vi "Coord window-Panel close handler.vi"   [LabVIEW 2017]
uses:
  Visualisation/Functional Imaging Viewer/SubVIs/Experiment header interface/Typedefs/Save-Load-Save as-Load last enum.ctl
  Globals/Coord window-Globals.vi
types:
  T1 = cluster{"Caption-Right button":string, "Caption-Left button":string, "Message to display":string, "Delay before close":u32, "Window Colour":u32, "Cancel button disabled?":enum8{"Enabled", "Disabled", "Disabled and Grayed Out"}}
  T2 = typedef "Coordinate list window refs.ctl" = cluster{"Window Name (i.e. Key)":string, "menu reference":refnum<k9>, "VI's reference":refnum<vi>, "Pane 1":refnum<vi>, "Pane 2":refnum<vi>, "Coord Listbox":refnum<vi>, "File name":refnum<vi>, "Picture Map":refnum<vi>, "Stage XYZ Position ind.":refnum<vi>}
  T3 = typedef "Save-Load-Save as-Load last enum.ctl" = enum16{"Save file", "Save file as", "Load file", "Load last file"}
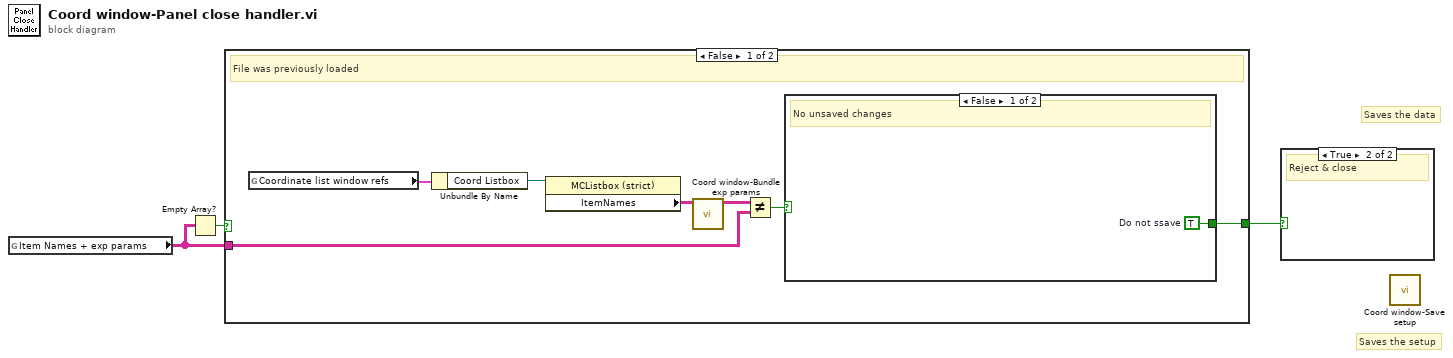
[diagram p0: block diagram]
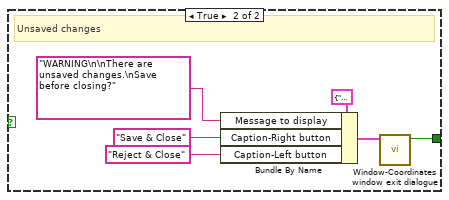
[diagram p2: hidden frame]
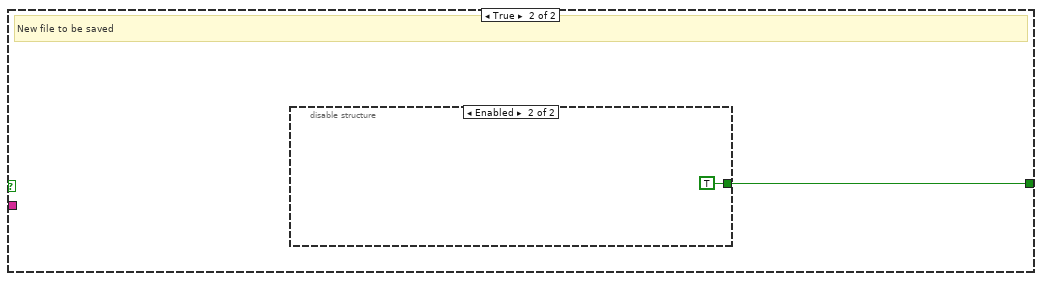
[diagram p3: hidden frame]
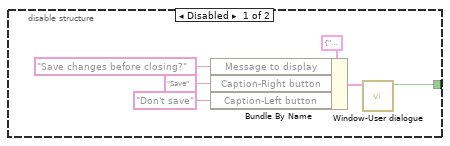
[diagram p4: hidden frame]
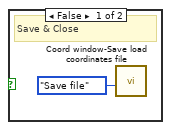
[diagram p5: hidden frame]
diagram:
  # "Saves the data"
  # "Saves the setup"
  n1 = global read "Coord window-Globals.vi" "Item Names + exp params"() -> (w2:string[][])
  n2 = Empty Array?(array=w2) -> (empty?=w1:bool)
  n3 = case shown="False" w1 {
    tunnel: [w6 w18] -> w3
    tunnel: w2 -> [w4 _]
    frame False {
      # "File was previously loaded"
      n4 = global read "Coord window-Globals.vi" "Coordinate list window refs"() -> (w10:T2)
      n5 = Unbundle By Name(w10) -> ("Coord Listbox"=w7:refnum<vi>)
      n6 = property on="Property Node" class="MCListbox (strict)"(reference=w7) -> ("ItemNames"=w8:string[][])  [unwired: 1 in, 2 out]
      n7 = call "Coord window-Bundle exp params.vi"("Item Names"=w8) -> ("Item Names + exp params"=w9:string[][])  [unwired: 10 in]
      n8 = Not Equal?(x=w9, y=w4) -> (x != y?=w5:bool)
      n9 = case shown="False" w5 {
        tunnel: [w11 w12] -> w6
        frame False {
          w11 = TRUE  # Do not ssave
          # "No unsaved changes"
        }
        frame True {
          # "Unsaved changes"
          n10 = Bundle By Name(cluster=T1 {"Caption-Right button"="Save", "Caption-Left button"="Cancel", "Message to display"="", "Delay before close"=0, "Window Colour"=16777226, "Cancel button disabled?"=enum."Enabled"} ("Input cluster"), "Message to display"="WARNING\n\nThere are unsaved changes.\nSave before closing?" ("Caption-Right button"), "Caption-Right button"="Save & Close", "Caption-Left button"="Reject & Close") -> (w17:T1)
          n11 = call "Window-Coordinates window exit dialogue.vi"("Input cluster"=w17) -> ("Left Button (Cancel)"=w12:bool)  [unwired: 10 in]
        }
      }
    }
    frame True {
      # "New file to be saved"
      n12 = disable-structure shown="Enabled" {
        disable-tunnel: [w19 TRUE ("Left Button (Cancel)")] -> w18
        frame Disabled {
          n13 = Bundle By Name(cluster=T1 {"Caption-Right button"="Save", "Caption-Left button"="Cancel", "Message to display"="", "Delay before close"=0, "Window Colour"=16777226, "Cancel button disabled?"=enum."Enabled"} ("Input cluster"), "Message to display"="Save changes before closing?" ("Caption-Right button"), "Caption-Right button"="Save", "Caption-Left button"="Don't save") -> (w24:T1)
          n14 = call "Window-User dialogue.vi"("Input cluster"=w24) -> ("Left Button (Cancel)"=w19:bool)  [unwired: 10 in]
        }
        frame Enabled {
        }
      }
    }
  }
  n15 = case shown="True" w3 {
    frame False {
      # "Save & Close"
      n16 = call "Coord window-Save load coordinates file.vi"("Function"=Save-Load-Save_as-Load_last_enum."Save file") -> ()  [unwired: 10 in, 1 out]
    }
    frame True {
      # "Reject & close"
    }
  }
  n17 = call "Coord window-Save setup.vi"() -> ()  [unwired: 11 in, 1 out]
